vi "blinkLED.vi"(8 "error in (no error)":errorcluster, 11 "LED in":refnum<class "LED.lvclass">) -> (0 "error out":errorcluster, 3 "LED out":refnum<class "LED.lvclass">)   [LabVIEW 2019, in "LED.lvclass"]
doc: "This method blinks the LED referenced in the InitializeLED method."
uses:
  LED.lvclass
  LED.lvclass/LED.ctl
  Sound/Sound.lvclass
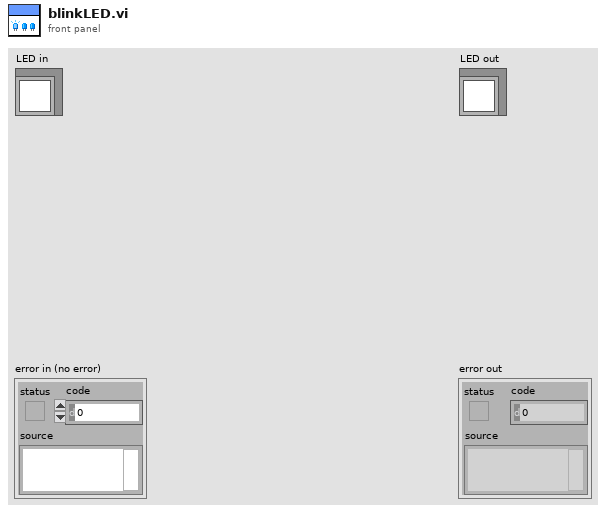
[diagram p1: front panel]
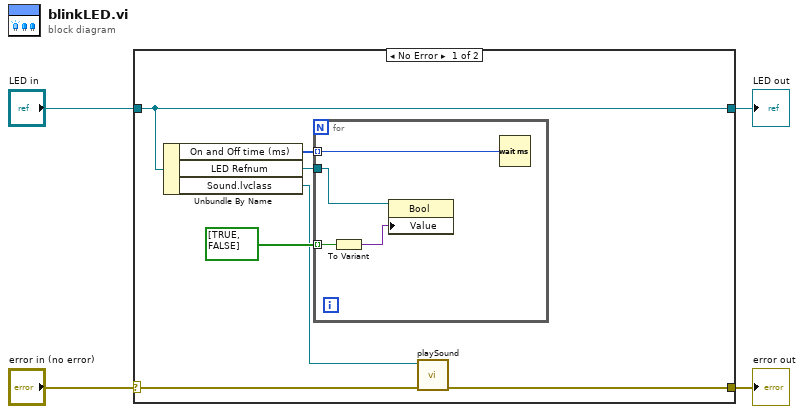
[diagram p0: block diagram]
diagram:
  n1 = case shown="No Error" "error in (no error)" {
    selector: "error in (no error)" -> [w11 w17]
    tunnel: [w7 w17] -> w3
    tunnel: [w10 w16] -> w1
    tunnel: "LED in" -> [w10 w16]
    frame No Error {
      n2 = Unbundle By Name(w10) -> ("On and Off time (ms)"=w5:u32[], "LED Refnum"=w8:refnum<vi>, "Sound.lvclass"=w6:refnum<class "Sound.lvclass">)
      n3 = for {
        tunnel: bool[] [TRUE, FALSE] -> [w15] mode=indexing
        tunnel: w8 -> [w13]
        tunnel: w5 -> [w14] mode=indexing
        n4 = To Variant(anything=w15) -> (Variant=w12:variant)
        n5 = property class="Bool"(reference=w13, "Value"=w12) -> ()  [unwired: 1 in, 2 out]
        n6 = Wait (ms)(milliseconds to wait=w14) -> ()  [unwired: 1 out]
      }
      n7 = call "playSound.vi"("error in (no error)"=w11, "Sound in"=w6) -> ("error out"=w7:errorcluster)  [unwired: 8 in, 1 out]
    }
    frame Error {
    }
  }
  "error out" <- w3
  "LED out" <- w1
